vi "ReadSharedVarU16.vi"(8 "entrée d'erreur (pas d'erreur)":errorcluster, 11 "refnum de variable partagée en entrée":refnum<k21>) -> (0 "sortie d'erreur":errorcluster, 2 "données en sortie":u16)   [LabVIEW 2013]
doc: "Ce VI permet d'ouvrir une variable partagée, d'y écrire un U16, et de la fermer. VI créé pour Open ModBus Eth 2.20 avec lesquel plusieurs variables partagées par le serveur OPC ne peuvent être ouvertes simultanément (ce qui était le cas avec la version 2.14)"
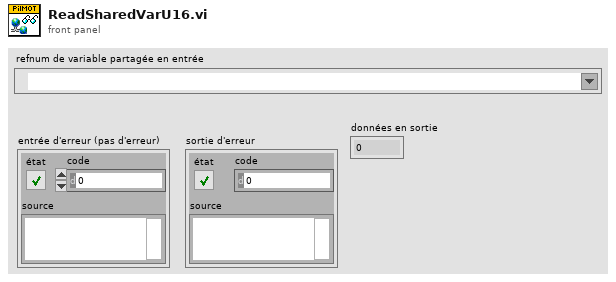
[diagram p1: front panel]
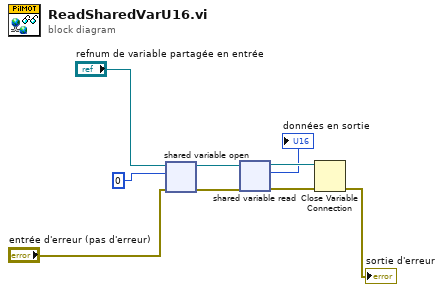
[diagram p0: block diagram]
diagram:
  n1 = shared-variable-open("refnum de variable partagée en entrée", "entrée d'erreur (pas d'erreur)", u16 0) -> (w4:refnum<k21>, w6:errorcluster)  [unwired: 1 in]
  n2 = shared-variable-read(w4, w6) -> (w3:refnum<k21>, w5:errorcluster, →"données en sortie":u16)  [unwired: 1 out]
  n3 = Close Variable Connection(8:w5, 11:w3) -> (0:→"sortie d'erreur":errorcluster)
